vi "QueryServer_AddQueryEvent.vi"(11 "gRPCid in":T1) -> (2 "QueryServer_Query":refnum<user-event>, 3 "gRPCid":T1)   [LabVIEW 2019, in "labview-grpc-query-server.lvlib"]
uses:
  labview-grpc-query-server.lvlib
  QueryServer_InvokeEventData.ctl
  VIs/grpcId.ctl
  QueryServer_QueryEventData.ctl
  a66ee327-264b-4784-bac1-fff8ba4a2692.vi
  VIs/gprc-support.lvlib
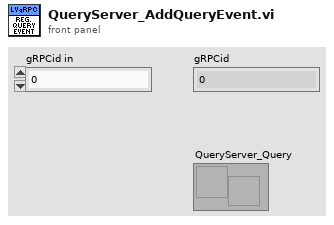
[diagram p1: front panel]
types:
  T1 = typedef "gprc-support.lvlib/grpcId.ctl" = u64
  T2 = typedef "labview-grpc-query-server.lvlib/QueryServer_QueryEventData.ctl" = cluster{"gRPCid":T1}
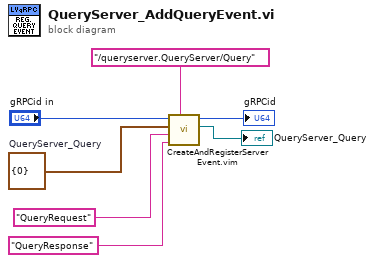
[diagram p0: block diagram]
diagram:
  w5 = T2 {"gRPCid"=0}  # QueryServer_Query
  n1 = call "CreateAndRegisterServerEvent.vim"("name"="/queryserver.QueryServer/Query", "Response Metadata Name"="QueryResponse" ("Name"), "Request Metadata Name"="QueryRequest" ("Name"), "event in"=w5, "gRPCid in"="gRPCid in") -> ("event"=→"QueryServer_Query":refnum<user-event>, "gRPCid"=→"gRPCid":T1)  [unwired: 5 in]
